vi "邻域去盲元-子VI.vi"(6 "error in":errorcluster, 8 "输入":dbl[][](array[numeric]), 10 "ãÐÖµ":dbl, 11 "尺寸":i32=5) -> (1 "中值滤波":dbl[][](array[numeric]), 3 "盲元表":dbl[][](array[numeric]), 4 "error out":errorcluster)   [LabVIEW 2016]
uses:
  <vilib>/Analysis/NI_AALBase.lvlib
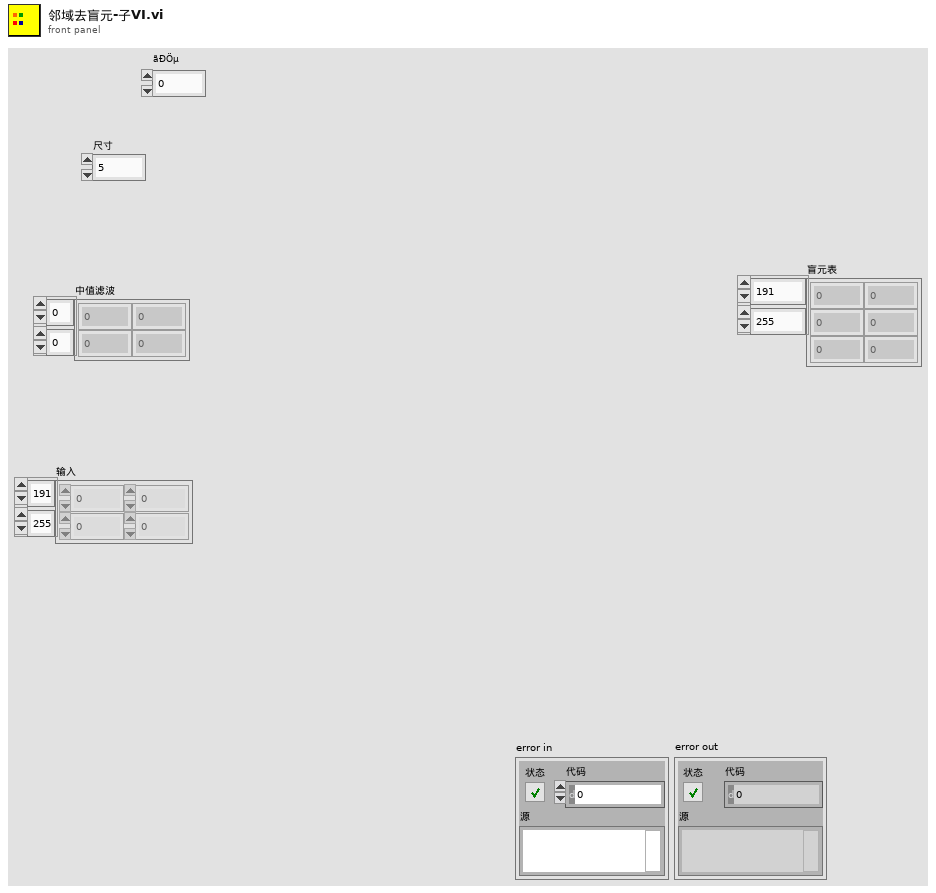
[diagram p1: front panel]
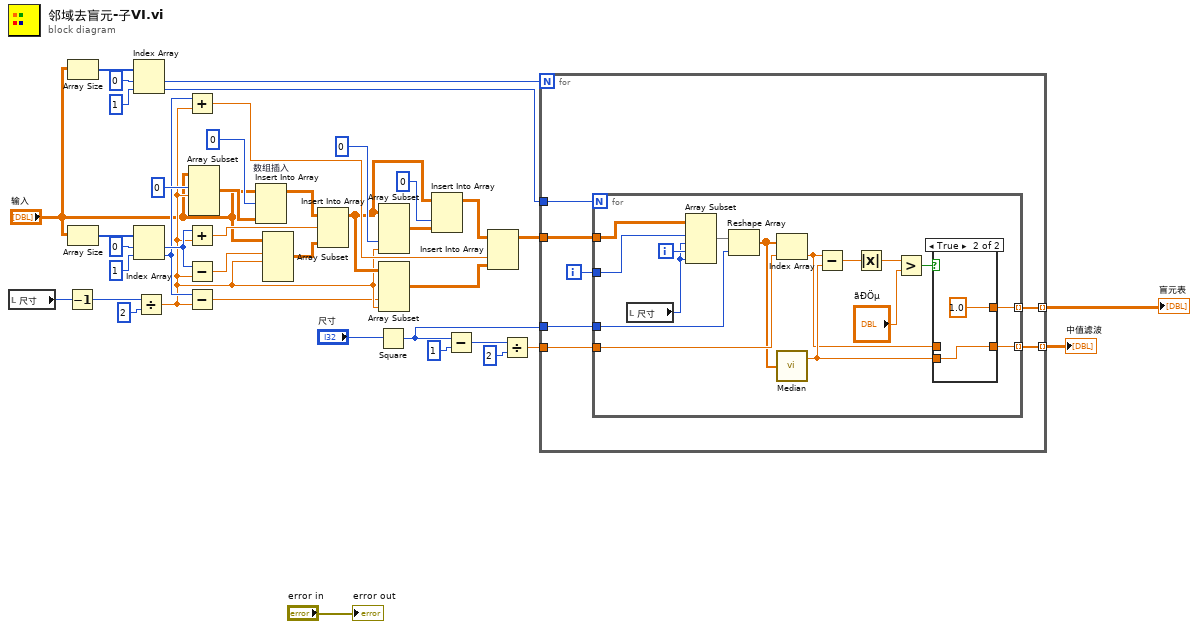
[diagram p0: block diagram]
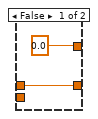
[diagram p2: hidden frame]
diagram:
  n1 = local read "尺寸"() -> (w24:i32)
  n2 = Decrement(x=w24) -> (x-1=w23:i32)
  n3 = Array Size(array="输入") -> (size(s)=w33:i32[])
  n4 = Array Size(array="输入") -> (size(s)=w11:i32[])
  n5 = Index Array(array=w33, index #1=0 ("索引"), index #2=1 ("索引")) -> (element #1=w30:i32, element #2=w29:i32)
  n6 = Index Array(array=w11, index #1=0 ("索引"), index #2=1 ("索引")) -> (element #1=w8:i32, element #2=w7:i32)
  n7 = Divide(x=w23, y=2) -> (x/y=w6:dbl)
  n8 = Add(x=w7, y=w6) -> (x+y=w20:dbl)
  n9 = Add(x=w8, y=w6) -> (x+y=w21:dbl)
  n10 = Subtract(x=w8, y=w6) -> (x-y=w18:dbl)
  n11 = Subtract(x=w7, y=w6) -> (x-y=w5:dbl)
  n12 = Array Subset(array="输入", index (row)=0 ("索引"), length (row)=w6) -> (w12:dbl[][])  [unwired: 2 in]
  n13 = Insert Into Array "数组插入"(array="输入", index (row)=0 ("索引 (行)"), new element=w12) -> (w27:dbl[][])  [unwired: 1 in]
  n14 = Array Subset(array="输入", index (row)=w18, length (row)=w6) -> (w17:dbl[][])  [unwired: 2 in]
  n15 = Insert Into Array(array=w27, index (row)=w21, new element=w17) -> (w14:dbl[][])  [unwired: 1 in]
  n16 = Square(x="尺寸") -> (x^2=w36:i32)
  n17 = Array Subset(array=w14, index (col)=0 ("索引"), length (col)=w6) -> (w15:dbl[][])  [unwired: 2 in]
  n18 = Array Subset(array=w14, index (col)=w5, length (col)=w6) -> (w13:dbl[][])  [unwired: 2 in]
  n19 = Insert Into Array(array=w14, index (col)=0 ("禁用的索引 (列)"), new element=w15) -> (w25:dbl[][])  [unwired: 1 in]
  n20 = Subtract(x=w36, y=1) -> (x-y=w39:i32)
  n21 = Insert Into Array(array=w25, index (col)=w20, new element=w13) -> (w3:dbl[][])  [unwired: 1 in]
  n22 = Divide(x=w39, y=2) -> (x/y=w37:dbl)
  n23 = for {
    N: w30 -> [_]
    tunnel: w3 -> [w47]
    tunnel: [w45] -> w35 mode=indexing
    tunnel: w36 -> [w44]
    tunnel: w37 -> [w43]
    tunnel: w29 -> [w42]
    tunnel: [w41] -> w1 mode=indexing
    i -> [w46]
    n24 = for {
      N: w42 -> [_]
      tunnel: w47 -> [w63]
      tunnel: w46 -> [w62]
      tunnel: [w60] -> w45 mode=indexing
      tunnel: w44 -> [w56]
      tunnel: w43 -> [w58]
      tunnel: [w48] -> w41 mode=indexing
      i -> [w61]
      n25 = local read "尺寸"() -> (w59:i32)
      n26 = Array Subset(array=w63, index (row)=w62, length (row)=w59, index (col)=w61, length (col)=w59) -> (w57:dbl[][])
      n27 = Reshape Array(w57, w56) -> (w55:dbl[])
      n28 = Index Array(array=w55, index=w58) -> (element=w50:dbl)
      n29 = call <vilib>:"Median.vi"("X"=w55) -> ("median"=w52:dbl)  [unwired: 1 out]
      n30 = Subtract(x=w50, y=w52) -> (x-y=w54:dbl)
      n31 = Absolute Value(x=w54) -> (abs(x)=w53:dbl)
      n32 = Greater?(x=w53, y="ãÐÖµ") -> (0:w51:bool)
      n33 = case shown="True" w51 {
        tunnel: w52 -> [_ w67]
        tunnel: [w65 w67] -> w60
        tunnel: w50 -> [w65 _]
        tunnel: [0.0 1.0] -> w48
        frame False {
        }
        frame True {
        }
      }
    }
  }
  "中值滤波" <- w35
  "盲元表" <- w1
  "error out" <- "error in"
